vi "Differential Pressure Release Valve Test.vi"(8 "error in (no error)":errorcluster, 11 "Context in":refnum<class "Context.lvclass">) -> (0 "error out":errorcluster, 3 "Context out":refnum<class "Context.lvclass">)   [LabVIEW 2016]
uses:
  Model/Model/Model.lvclass
  States/State/State.lvclass
  Context.lvclass
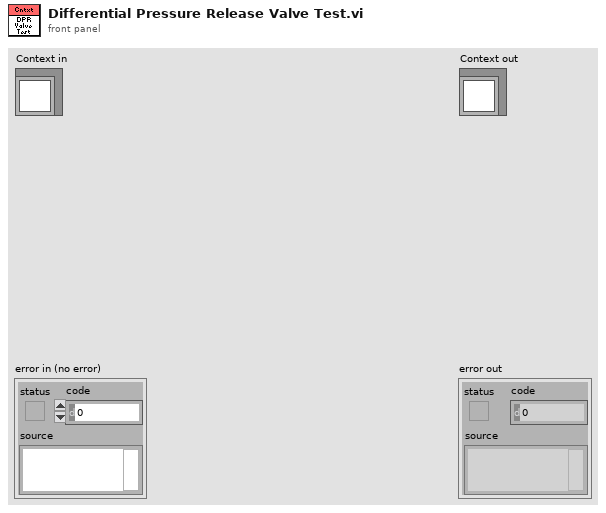
[diagram p1: front panel]
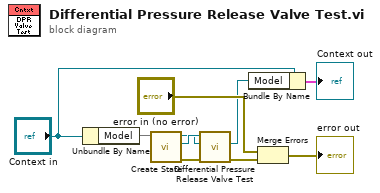
[diagram p0: block diagram]
diagram:
  n1 = Unbundle By Name("Context in") -> ("Model"=w10)
  n2 = call "Create State.vi"("Model in"=w10) -> ("error out"=w1:errorcluster, "State"=w5:refnum<class "State.lvclass">, "Model out"=w4:refnum<class "Model.lvclass">)  [unwired: 8 in]
  n3 = call-dynamic "Differential Pressure Release Valve Test.vi"("error in (no error)"=w1, "Model in"=w4, "State in"=w5) -> ("error out"=w2:errorcluster, "Model out"=w3:refnum<class "Model.lvclass">)  [unwired: 6 in, 1 out]
  n4 = Bundle By Name(cluster="Context in", "Model"=w3) -> (→"Context out":cluster{})
  n5 = Merge Errors("error in (no error)", w2) -> (→"error out":errorcluster)
